vi "LeCroy.Close Session.vi"(8 "Error In":errorcluster, 11 "LeCroy.Session in":T1) -> (0 "Error Out":errorcluster)   [LabVIEW 2018]
uses:
  typedefs/LeCroy.Session.ctl
  Driver/lecroy_wave_series/LeCroy Wave Series/LeCroy Wave Series.lvlib
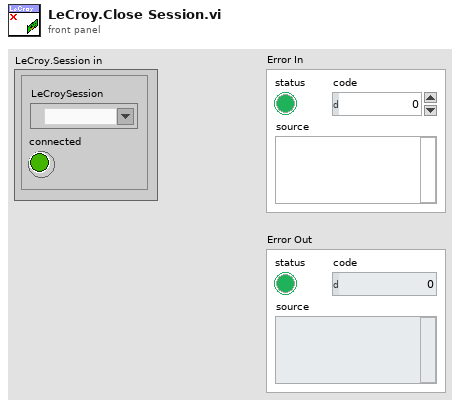
[diagram p1: front panel]
types:
  T1 = typedef "LeCroy.Session.ctl" = cluster{"LeCroySession":refnum<visa-resource-name>, "connected":bool}
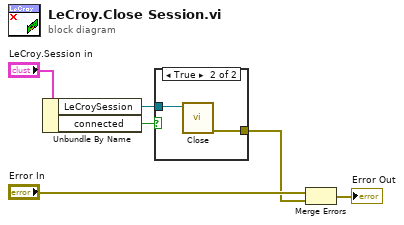
[diagram p0: block diagram]
diagram:
  n1 = Unbundle By Name("LeCroy.Session in") -> ("LeCroySession"=w2:refnum<visa-resource-name>, "connected"=w1:bool)
  n2 = case shown="True" w1 {
    tunnel: [_ w8] -> w4
    tunnel: w2 -> [_ w7]
    frame False {
    }
    frame True {
      n3 = call "Close.vi"("VISA resource name"=w7) -> ("error out"=w8:errorcluster)  [unwired: 10 in]
    }
  }
  n4 = Merge Errors("Error In", w4) -> (→"Error Out":errorcluster)
